vi "System_KillProcess.vi"(8 "Error In":errorcluster, 11 "Task Name":string) -> (0 "Error Out":errorcluster)   [LabVIEW 2017]
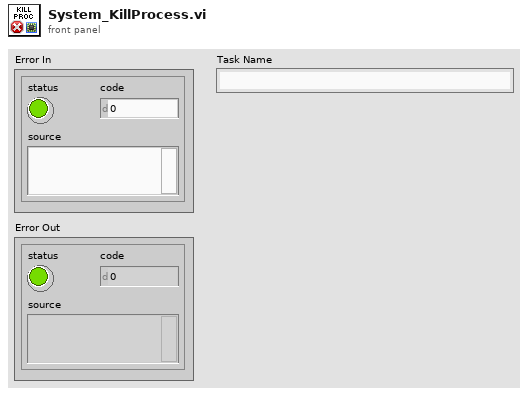
[diagram p1: front panel]
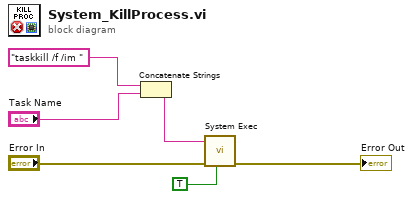
[diagram p0: block diagram]
diagram:
  n1 = Concatenate Strings("taskkill /f /im " ("string"), "Task Name") -> (w4:string)
  n2 = call <vilib>:"System Exec.vi"("run minimized? (F)"=TRUE, "error in (no error)"="Error In", "command line"=w4) -> ("error out"=→"Error Out":errorcluster)  [unwired: 5 in, 3 out]
